vi "Read port.vi"(8 "error in (no error)":errorcluster, 11 "Database Manager in":refnum<class "Database Manager.lvclass">) -> (0 "error out":errorcluster, 2 "port":i32, 3 "Database Manager out":refnum<class "Database Manager.lvclass">)   [LabVIEW 2021, in "Database Manager.lvclass"]
uses:
  Database Manager.lvclass
  Database Manager.lvclass/Database Manager.ctl
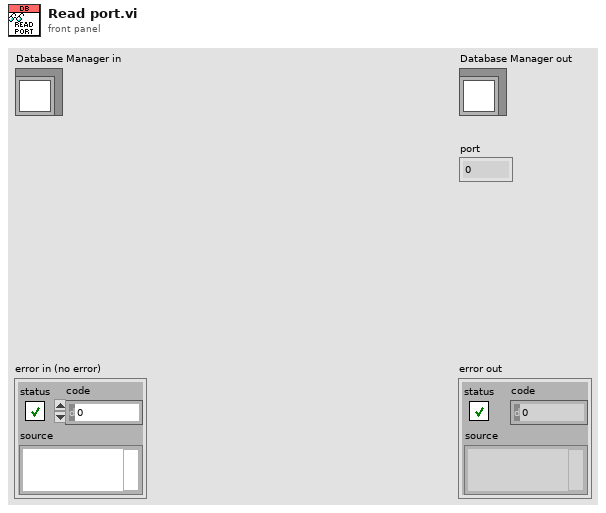
[diagram p1: front panel]
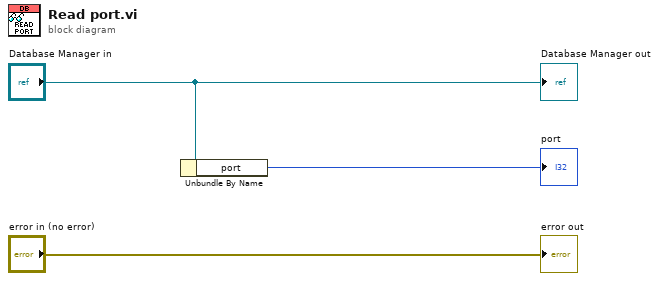
[diagram p0: block diagram]
diagram:
  n1 = Unbundle By Name("Database Manager in") -> ("port"=→"port":i32)
  "error out" <- "error in (no error)"
  "Database Manager out" <- "Database Manager in"
